vi "Flaps_AntiBack.vi"(2 "Toggle":bool, 3 "MtrPwrIn":dbl) -> (1 "MtrPwrOut":dbl)   [LabVIEW 2017]
uses:
  <vilib>/Rock Robotics/WPI/Solenoid/Deprecated/WPI_SolenoidSetBool.vi
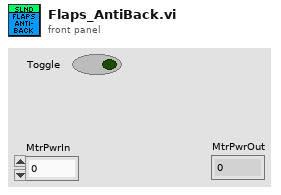
[diagram p1: front panel]
types:
  T1 = typedef "WPI_SolenoidDevRef.ctl" = cluster{"DevStatus":errorcluster, "Pneumatics Control Module":u8, "Forward Solenoid Channel":T2, "Reverse Solenoid Channel":T2}
  T2 = typedef "WPI_SolenoidChannel.ctl" = enum8{"Solenoid 0", "Solenoid 1", "Solenoid 2", "Solenoid 3", "Solenoid 4", "Solenoid 5", "Solenoid 6", "Solenoid 7", "Invalid"}
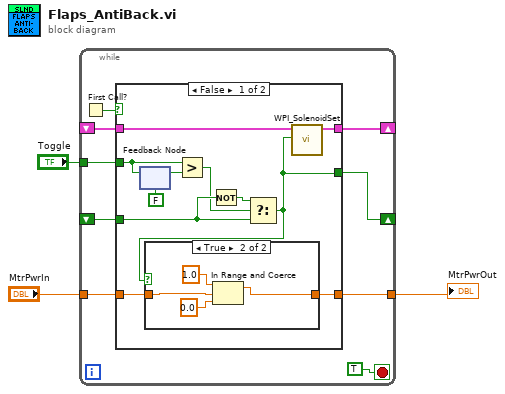
[diagram p0: block diagram]
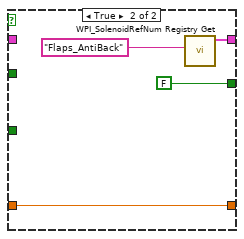
[diagram p3: hidden frame]
diagram:
  n1 = while {
    shift-right: [w9] -> _
    shift-left: _ -> [w10]
    shift-right: [w8] -> _
    shift-left: _ -> [w7]
    tunnel: "Toggle" -> [w6]
    tunnel: "MtrPwrIn" -> [w5]
    tunnel: [w4] -> w1
    stop <- TRUE stop-if-true
    n2 = First Call?() -> (First Call?: T/F=w11:bool)
    n3 = case shown="False" w11 {
      tunnel: w10 -> [w20 _]
      tunnel: [w13 FALSE ("Shift")] -> w9
      tunnel: [w22 w31] -> w8
      tunnel: w7 -> [w23 _]
      tunnel: w6 -> [w17 _]
      tunnel: w5 -> [w15 w29]
      tunnel: [w14 w29] -> w4
      frame False {
        n4 = feedback #1(FALSE) -> (w19:bool)
        n5 = feedback-in #1(w17) -> ()
        n6 = Greater?(x=w17, y=w19) -> (0:w16:bool)
        n7 = Not(x=w20) -> (.not. x?=w21:bool)
        n8 = Select(t=w21, s=w16, f=w20) -> (s? t:f=w13:bool)
        n9 = case shown="True" w13 {
          tunnel: w15 -> [w24 w26]
          tunnel: [w24 w25] -> w14
          frame False {
          }
          frame True {
            n10 = In Range and Coerce(upper limit=1.0, x=w26, lower limit=0.0) -> (coerced(x)=w25:dbl)  [unwired: 1 out]
          }
        }
        n11 = call-poly <vilib>:"WPI_SolenoidSet.vi"("Value"=w13, "SolenoidDevRef"=w23) -> ("SolenoidDevRef"=w22:T1)  [unwired: 8 in, 1 out]
      }
      frame True {
        n12 = call <vilib>:"WPI_SolenoidRefNum Registry Get.vi"("refnum name"="Flaps_AntiBack") -> ("SolenoidDevRef"=w31:T1)  [unwired: 9 in, 1 out]
      }
    }
  }
  "MtrPwrOut" <- w1
